vi "Split and Merge.vi"(10 "Split Threshold":dbl=20.0, 11 "Line":T1) -> (0 "Line Graph":cluster{dbl[], dbl[]}[](graph), 2 "Lines":T1[](array[typedef]), 3 "Corners":T2[](array[typedef]))   [LabVIEW 2017]
uses:
  Vector Library/Line.ctl
  Vector Library/Vector.ctl
panel:
  out "Merge":cluster{dbl[], dbl[]}[](graph)
  out "Split":cluster{dbl[], dbl[]}[](graph)
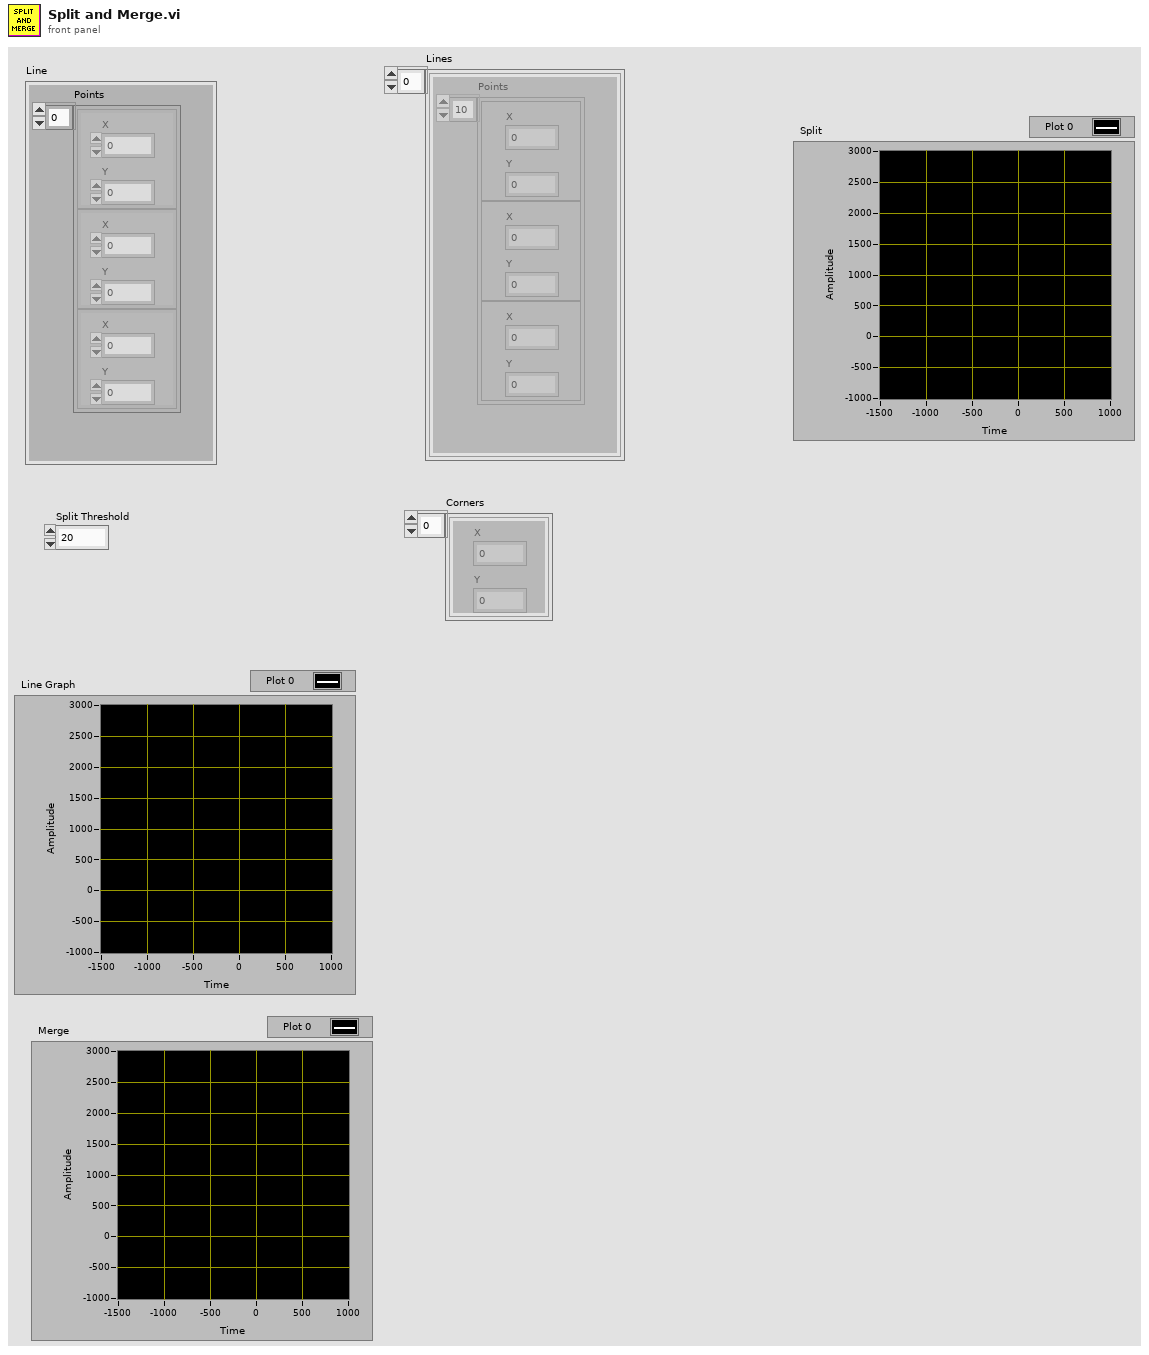
[diagram p1: front panel]
types:
  T1 = typedef "Line.ctl" = cluster{"Points":T2[]}
  T2 = typedef "Vector.ctl" = cluster{"X":dbl, "Y":dbl}
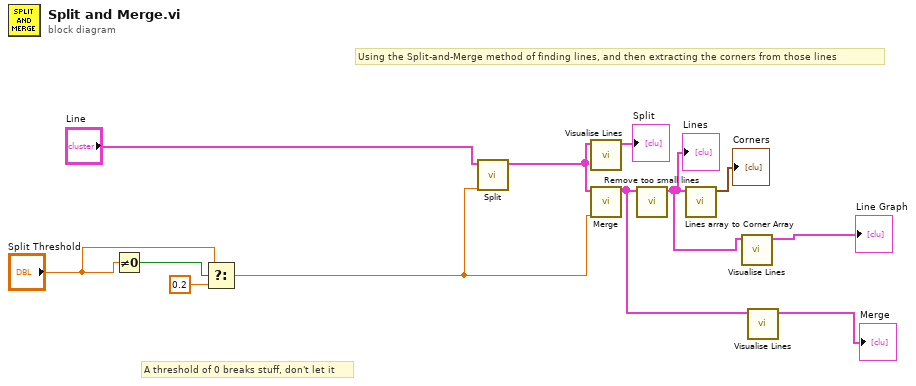
[diagram p0: block diagram]
diagram:
  # "A threshold of 0 breaks stuff, don't let it"
  # "Using the Split-and-Merge method of finding lines, and then extracting the corners from those lines"
  n1 = Not Equal To 0?(x="Split Threshold") -> (x != 0?=w8:bool)
  n2 = Select(t="Split Threshold", s=w8, f=0.2) -> (s? t:f=w5:dbl)
  n3 = call "Split.vi"("Split Threshold"=w5, "Original Line"="Line") -> ("Resulting Lines"=w11:T1[])  [unwired: 9 in]
  n4 = call "Visualise Lines.vi"("Lines"=w11) -> ("XY Graph"=→"Split":cluster{dbl[], dbl[]}[])  [unwired: 10 in]
  n5 = call "Merge.vi"("Merge Threshold"=w5, "Original Lines"=w11) -> ("Merged Lines"=w1:T1[])  [unwired: 9 in]
  n6 = call "Remove too small lines.vi"("All Lines"=w1) -> ("Big Enough Lines"=w3:T1[])  [unwired: 10 in]
  "Lines" <- w3
  n7 = call "Lines array to Corner Array.vi"("Lines"=w3) -> ("Corners"=→"Corners":T2[])  [unwired: 10 in]
  n8 = call "Visualise Lines.vi"("Lines"=w3) -> ("XY Graph"=→"Line Graph":cluster{dbl[], dbl[]}[])  [unwired: 10 in]
  n9 = call "Visualise Lines.vi"("Lines"=w1) -> ("XY Graph"=→"Merge":cluster{dbl[], dbl[]}[])  [unwired: 10 in]
